vi "UpdateSomeButtons.vi"(1 "Load":refnum<vi>, 2 "Destination:":path, 3 "error in (no error)":errorcluster, 4 "Store Data":bool) -> (5 "error":errorcluster)   [LabVIEW 2009]
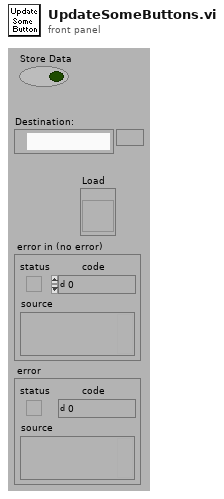
[diagram p1: front panel]
types:
  T1 = enum16{"read/write", "read-only", "write-only", "write-only (truncate)"}
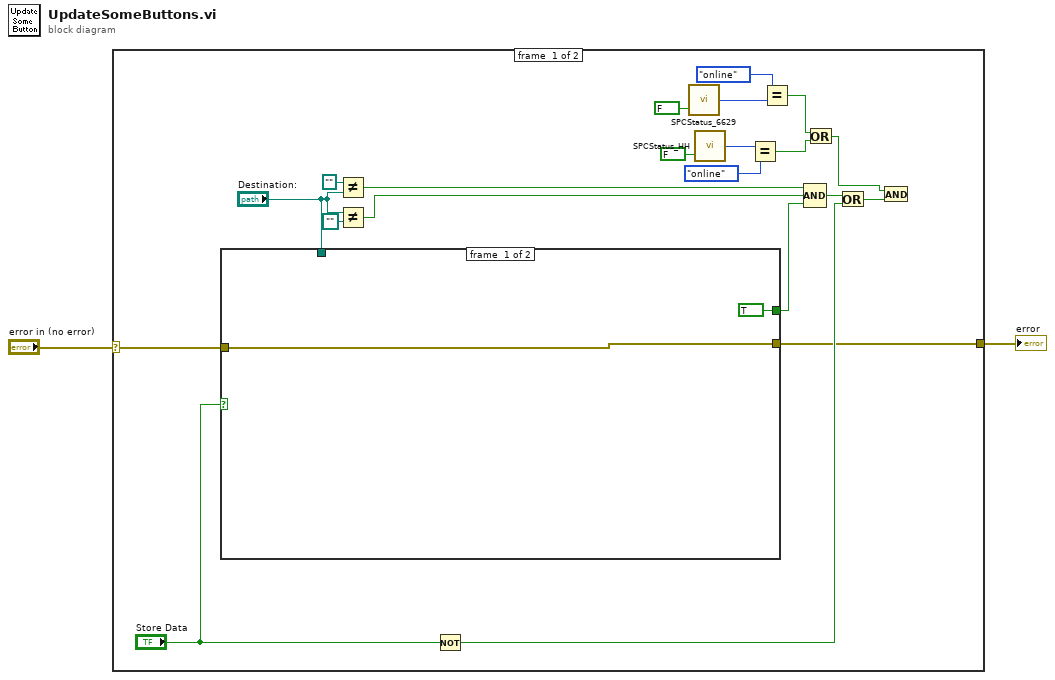
[diagram p0: block diagram]
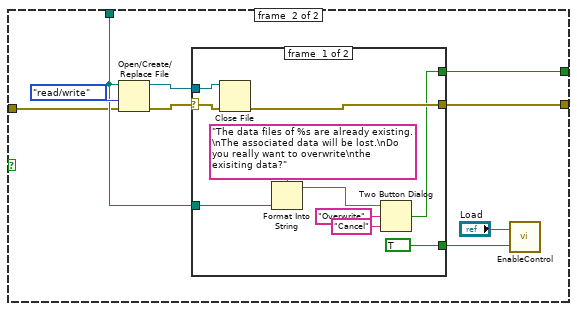
[diagram p2: hidden frame]
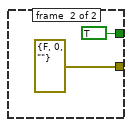
[diagram p3: hidden frame]
diagram:
  n1 = case shown="No Error" "error in (no error)" {
    selector: "error in (no error)" -> [w15 w47]
    tunnel: [w14 w47] -> w1
    frame #0 {
      n2 = case shown="True" "Store Data" {
        tunnel: "Destination:" -> [_ w32]
        tunnel: w15 -> [w25 w31]
        tunnel: [w25 w30] -> w14
        tunnel: [TRUE ("T button?") w27] -> w12
        frame #0 {
        }
        frame #1 {
          n3 = Open/Create/Replace File(file path (use dialog)=w32, error in=w31, access (0:read/write)=T1."read/write" ("open mode (0)")) -> (refnum out=w33:refnum<file>, error out=w28:errorcluster)  [unwired: 3 in, 1 out]
          n4 = case shown="No Error" w28 {
            selector: w28 -> [w37 _]
            tunnel: w33 -> [w44 _]
            tunnel: w32 -> [w42 _]
            tunnel: [w38 errorcluster {"status"=FALSE, "code"=0, "source"=""} ("error out")] -> w30
            tunnel: [w36 TRUE ("T button?")] -> w27
            tunnel: [TRUE _] -> w26
            frame #0 {
              n5 = Close File(refnum=w44, error in=w37) -> (error out=w38:errorcluster)  [unwired: 1 out]
              n6 = Format Into String(format string="The data files of %s are already existing.\nThe associated data will be lost.\nDo you really want to overwrite\nthe exisiting data?", w42) -> (resulting string=w41:string)  [unwired: 2 in, 1 out]
              n7 = Two Button Dialog(message=w41, 1:"Cancel" ("F button name (\"Cancel\")"), 2:"Overwrite" ("T button name (\"OK\")")) -> (T button?=w36:bool)
            }
            frame #1 {
            }
          }
          n8 = call "EnableControl.vi"("Enable"=w26, "Reference"="Load") -> ()
        }
      }
      n9 = Not Equal?(x=path "" ("Empty Path Constant"), y="Destination:") -> (x != y?=w19:bool)
      n10 = Not Equal?(x="Destination:", y=path "" ("Not A Path Constant")) -> (x != y?=w18:bool)
      n11 = Not(x="Store Data") -> (.not. x?=w23:bool)
      n12 = call "SPCStatus_6629.vi"("Set/Get"=FALSE) -> ("Status (output)"=w11:enum16{"offline", "online", "busy"})  [unwired: 1 in]
      n13 = call "SPCStatus_HH.vi"("Set/Get"=FALSE) -> ("Status (output)"=w9:enum16{"offline", "online", "busy"})  [unwired: 1 in]
      n14 = Equal?(x=w9, y=enum16{"offline", "online", "busy"}."online") -> (x = y?=w6:bool)
      n15 = Equal?(x=enum16{"offline", "online", "busy"}."online", y=w11) -> (x = y?=w8:bool)
      n16 = Compound Arithmetic op=AND(w19, w18, w12) -> (w17:bool)
      n17 = Or(x=w8, y=w6) -> (x .or. y?=w5:bool)
      n18 = Or(x=w17, y=w23) -> (x .or. y?=w22:bool)
      n19 = And(x=w5, y=w22) -> ()  [unwired: 1 out]
    }
    frame #1 {
    }
  }
  "error" <- w1
